vi "2023 actual arm2.vi"(8 "y (final pt)":dbl, 9 "x (final pt)":dbl, 10 "length 2nd arm":dbl, 11 "length 1st arm":dbl) -> (0 "y1c2 (1st arm)":dbl, 1 "x1c2 (1st arm)":dbl, 2 "y1c1 (1st arm)":dbl, 3 "x1c1 (1st arm)":dbl)   [LabVIEW 2023]
panel:
  out "Array":bool[](array[boolean])
  out "y increment":dbl
  out "x increment":dbl
  in  "intial y":dbl
  in  "initial x":dbl
  in  "iterations":dbl
  out "p1 (for debug":dbl
  out "q2 (config 1)":dbl
  out "q2 (config 2)":dbl
  out "q1 (config 2)":dbl
  out "x1c2 (2nd arm)":dbl
  out "y1c2 (2nd arm)":dbl
  out "y1c1 (2nd arm)":dbl
  out "x1c1 (2nd arm)":dbl
  out "q1 (config 1)":dbl
  out "a2 (for debug)":dbl
  out "Configuration 2":cluster{"X":dbl, "Y":dbl}[](graph)
  out "Configuration 1":cluster{"X":dbl, "Y":dbl}[](graph)
  # "angles (q's) in radians"
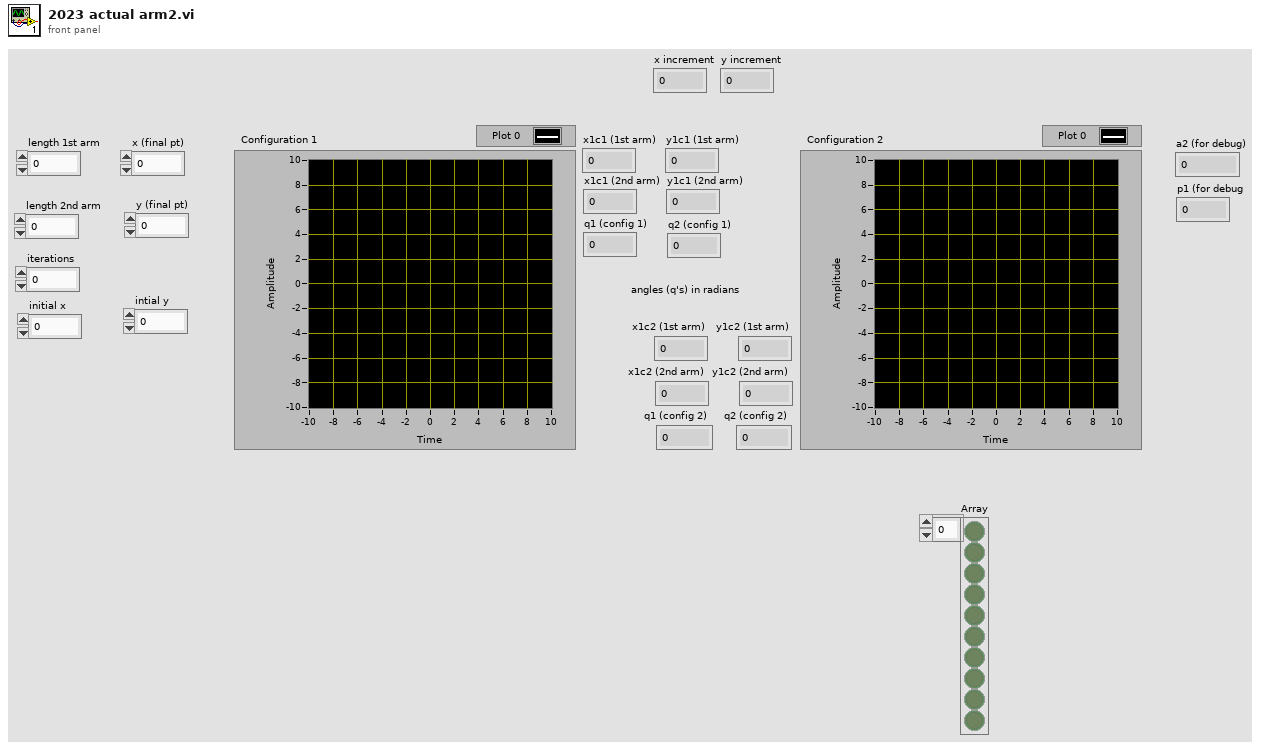
[diagram p1: front panel]
types:
  T1 = cluster{"x1 graph (2nd arm)":dbl, "y1 graph (2nd arm)":dbl}
  T2 = cluster{"x1 graph (2nd arm)":dbl, "y1 graph (2nd arm)":dbl}[]
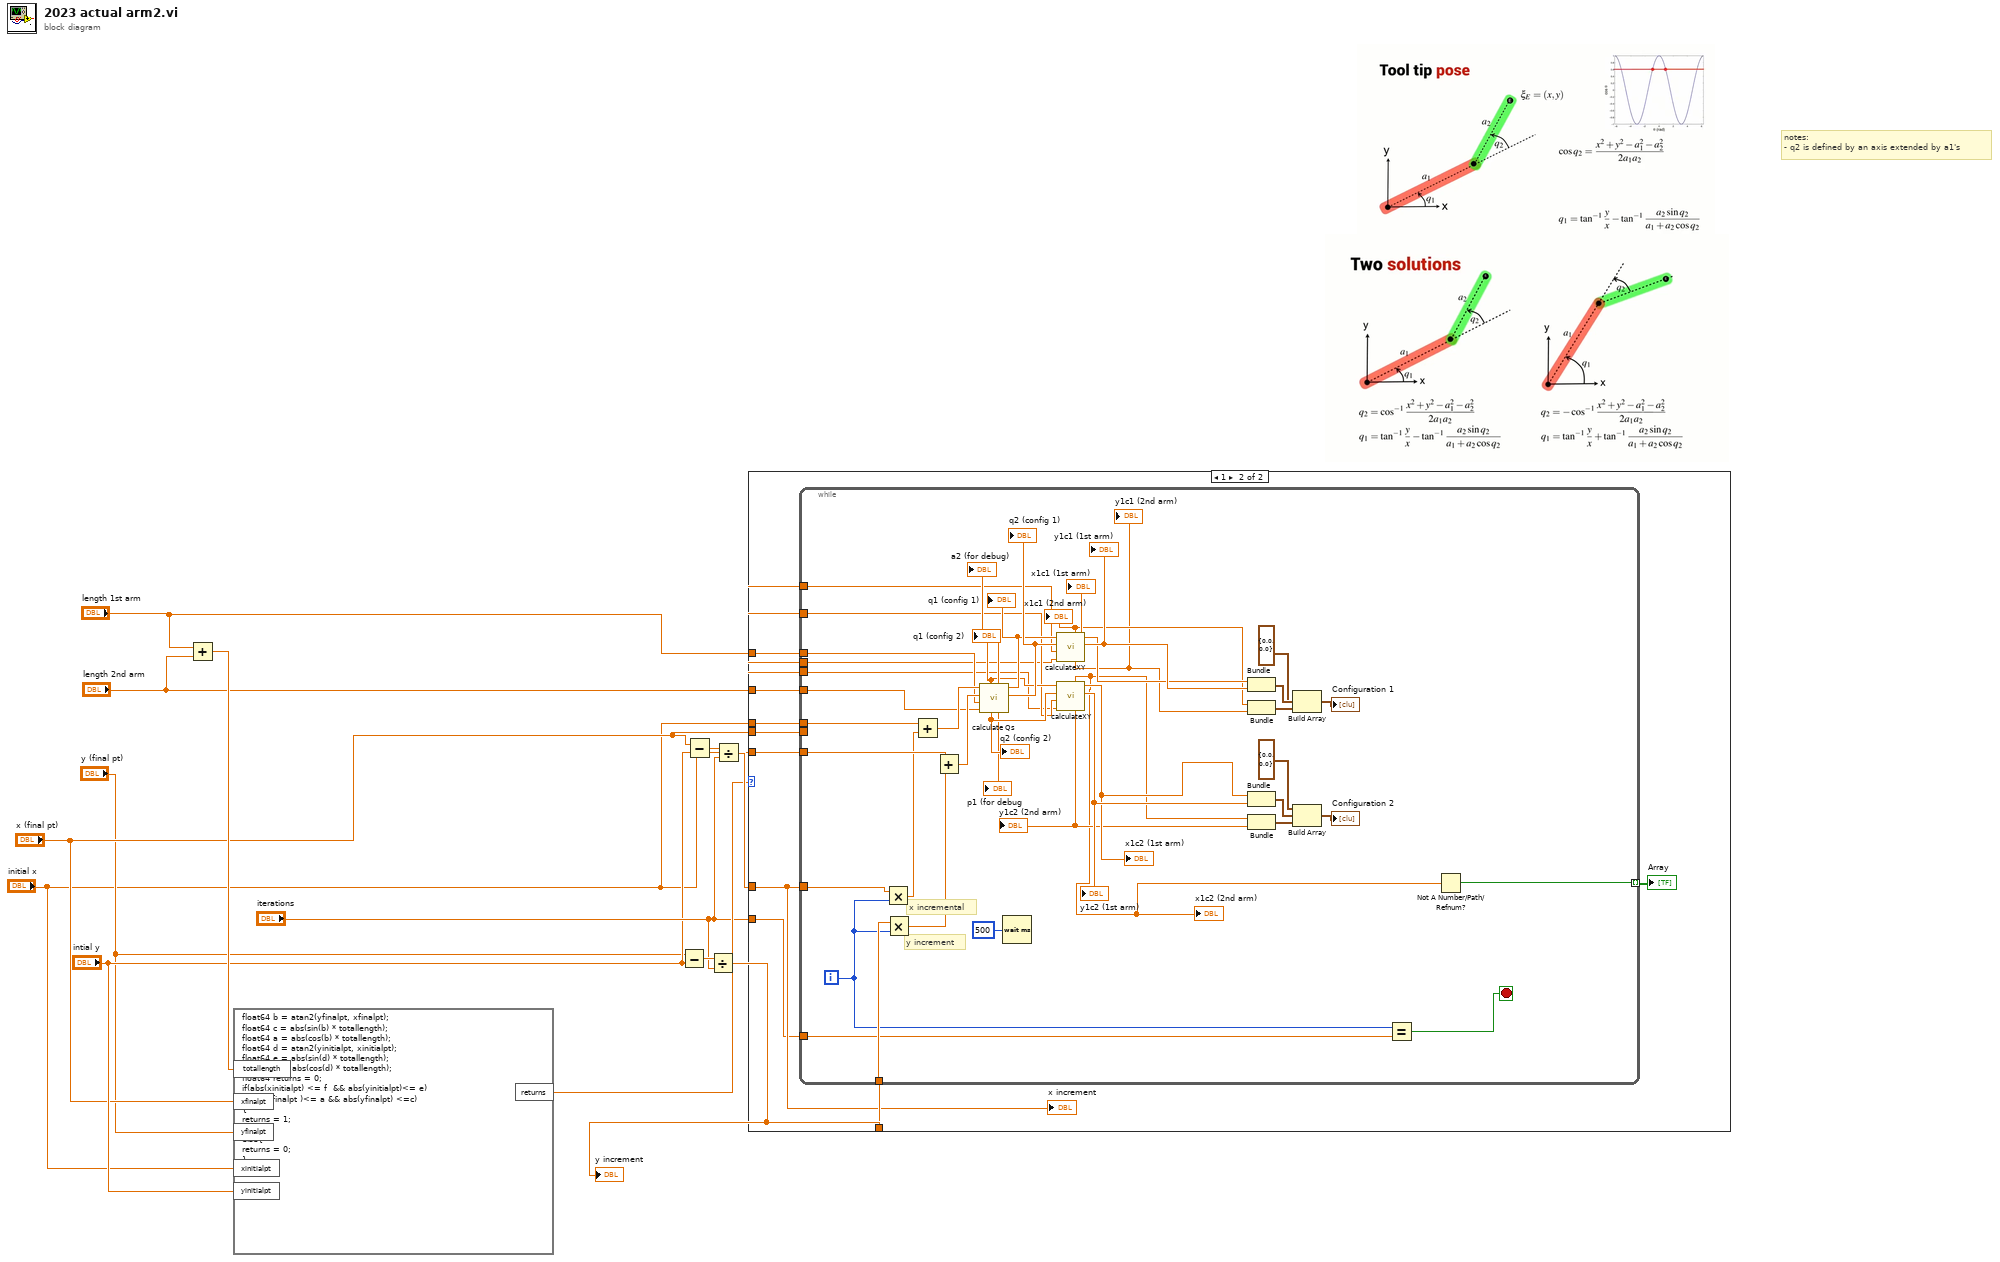
[diagram p0: block diagram]
diagram:
  # "notes:\n- q2 is defined by an axis extended by a1's"
  n1 = Add(x="length 1st arm", y="length 2nd arm") -> (x+y=w9:dbl)
  n2 = formula code="float64 b = atan2(yfinalpt, xfinalpt);\nfloat64 c = abs(sin(b) * totallength);\nfloat64 a = abs(cos(b) * totallength);\nfloat64 d = atan2(yinitialpt, xinitialpt);\nfloat64 e = abs(sin(d) * totallength);\nfloat64 f =  abs(cos(d) * totallength);\nfloat64 returns = 0;\nif(abs(xinitialpt) <= f  && abs(yinitialpt)<= e)\nif(abs(xfinalpt )<= a && abs(yfinalpt) <=c)\n{\nreturns = 1;\n}\nelse{\nreturns = 0;\n}"("totallength"=w9, "xfinalpt"="x (final pt)", "yfinalpt"="y (final pt)", "xinitialpt"="initial x", "yinitialpt"="intial y") -> ("returns"=w8:dbl)
  n3 = Subtract(x="y (final pt)", y="intial y") -> (x-y=w13:dbl)
  n4 = Subtract(x="x (final pt)", y="initial x") -> (x-y=w12:dbl)
  n5 = Divide(x=w13, y="iterations") -> (x/y=w11:dbl)
  "y increment" <- w11
  n6 = Divide(x=w12, y="iterations") -> (x/y=w10:dbl)
  n7 = case shown="1" w8 {
    tunnel: w11 -> [_ w22]
    tunnel: w10 -> [_ w21]
    tunnel: "length 1st arm" -> [_ w20]
    tunnel: "length 2nd arm" -> [_ w19]
    tunnel: "x (final pt)" -> [_ w18]
    tunnel: "initial x" -> [_ w17]
    tunnel: "intial y" -> [_ w16]
    tunnel: "iterations" -> [_ w15]
    frame 0, Default {
    }
    frame 1 {
      n8 = while {
        tunnel: w18 -> [_]
        tunnel: w22 -> [w45]
        tunnel: w21 -> [w44]
        tunnel: w16 -> [w42]
        tunnel: w17 -> [w41]
        tunnel: w20 -> [w35]
        tunnel: w20 -> [w34]
        tunnel: w20 -> [w33]
        tunnel: w19 -> [w32]
        tunnel: w19 -> [w31]
        tunnel: w19 -> [w30]
        tunnel: w15 -> [w26]
        tunnel: [w23] -> w14 mode=indexing
        i -> [w27]
        stop <- w25 stop-if-true
        # "x incremental"
        # "y increment"
        n9 = Multiply(x=w44, y=w27) -> (x*y=w40:dbl)
        n10 = Multiply(x=w45, y=w27) -> (x*y=w43:dbl)
        n11 = Add(x=w41, y=w40) -> (x+y=w39:dbl)
        n12 = Add(x=w42, y=w43) -> (x+y=w38:dbl)
        n13 = call "calculate Qs.vi"("length 2"=w32, "length 1"=w35, "y"=w38, "x"=w39) -> ("q2 (config 1)"=w53:dbl, "q1 (config 1)"=w51:dbl, "p1 (for debug"=→"p1 (for debug":dbl, "a2 (for debug)"=→"a2 (for debug)":dbl, "q2 (config 2)"=w54:dbl, "q1 (config 2)"=w50:dbl)  [unwired: 2 out]
        "q1 (config 1)" <- w51
        "q1 (config 2)" <- w50
        "q2 (config 2)" <- w54
        "q2 (config 1)" <- w53
        n14 = Wait (ms)(milliseconds to wait=u32 500) -> ()  [unwired: 1 out]
        n15 = call "calculateXY.vi"("q1"=w51, "q2"=w53, "length 1"=w33, "length 2"=w30) -> ("x1 graph (2nd arm)"=w37:dbl, "y1 graph (2nd arm)"=w29:dbl, "x1 (1st arm)"=w46:dbl, "y1 (1st arm)"=w62:dbl)  [unwired: 1 in, 2 out]
        "x1c1 (2nd arm)" <- w37
        "x1c1 (1st arm)" <- w46
        "y1c1 (1st arm)" <- w62
        "y1c1 (2nd arm)" <- w29
        n16 = call "calculateXY.vi"("q1"=w50, "q2"=w54, "length 1"=w34, "length 2"=w31) -> ("x1 graph (2nd arm)"=w24:dbl, "y1 graph (2nd arm)"=w28:dbl, "x1 (1st arm)"=w48:dbl, "y1 (1st arm)"=w55:dbl)  [unwired: 1 in, 2 out]
        "x1c2 (1st arm)" <- w48
        "y1c2 (1st arm)" <- w55
        "y1c2 (2nd arm)" <- w28
        "x1c2 (2nd arm)" <- w24
        n17 = Bundle("x1 (1st arm)"=w46, "y1 (1st arm)"=w62) -> (w61:cluster{"x1 (1st arm)":dbl, "y1 (1st arm)":dbl})  [unwired: 1 in]
        n18 = Bundle("x1 graph (2nd arm)"=w37, "y1 graph (2nd arm)"=w29) -> (w60:T1)  [unwired: 1 in]
        n19 = Bundle("x1 (1st arm)"=w48, "y1 (1st arm)"=w55) -> (w57:cluster{"x1 (1st arm)":dbl, "y1 (1st arm)":dbl})  [unwired: 1 in]
        n20 = Bundle("x1 graph (2nd arm)"=w24, "y1 graph (2nd arm)"=w28) -> (w47:T1)  [unwired: 1 in]
        n21 = Build Array(cluster{dbl, dbl} {0.0, 0.0} ("element"), w61, w60) -> (→"Configuration 1":T2)
        n22 = Build Array(cluster{dbl, dbl} {0.0, 0.0} ("element"), w57, w47) -> (→"Configuration 2":T2)
        n23 = Equal?(x=w27, y=w26) -> (x = y?=w25:bool)
        n24 = Not A Number/Path/Refnum?(number/path/refnum=w24) -> (NaN/Path/Refnum?=w23:bool)
      }
      "Array" <- w14
      "x increment" <- w21
    }
  }
